vi "Update Graph Plots.vi"(11 "UI Data in":refnum<class "Settings UI.lvclass">) -> (3 "UI Data out":refnum<class "Settings UI.lvclass">)   [LabVIEW 2020, in "Output Sequencer.lvlib" / "Settings UI.lvclass"]
uses:
  Settings UI.lvclass
  Settings UI.lvclass/Settings UI.ctl
  Output Sequencer/Globals/Global Strings.vi
  Output Sequencer/Output Sequencer.lvclass
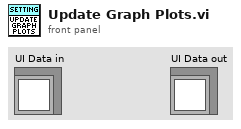
[diagram p1: front panel]
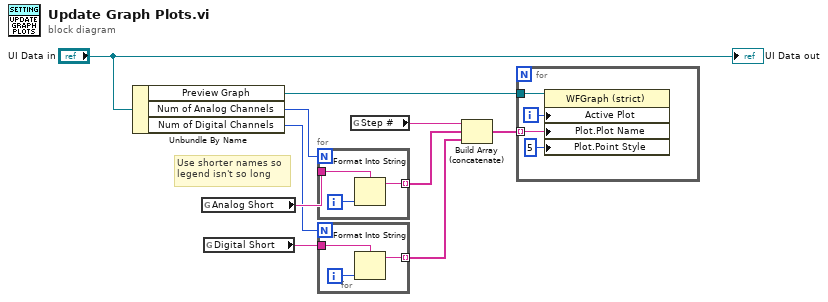
[diagram p0: block diagram]
diagram:
  # "Use shorter names so\nlegend isn't so long"
  n1 = Unbundle By Name("UI Data in") -> ("Preview Graph"=w4:refnum<vi>, "Num of Analog Channels"=w9:i32, "Num of Digital Channels"=w2:i32)
  n2 = global read "Global Strings.vi" "Analog Short"() -> (w5:string)
  n3 = global read "Global Strings.vi" "Digital Short"() -> (w3:string)
  n4 = for {
    N: w9 -> [_]
    tunnel: w5 -> [w12]
    tunnel: [w11] -> w6 mode=indexing
    i -> [w13]
    n5 = Format Into String(format string=w12, w13) -> (resulting string=w11:string)  [unwired: 2 in, 1 out]
  }
  n6 = for {
    N: w2 -> [_]
    tunnel: w3 -> [w15]
    tunnel: [w14] -> w1 mode=indexing
    i -> [w16]
    n7 = Format Into String(format string=w15, w16) -> (resulting string=w14:string)  [unwired: 2 in, 1 out]
  }
  n8 = global read "Global Strings.vi" "Step #"() -> (w7:string)
  n9 = Build Array (concatenate)(w7, w6, w1) -> (w8:string[])
  n10 = for {
    tunnel: w8 -> [w19] mode=indexing
    tunnel: w4 -> [w17]
    i -> [w20]
    n11 = property class="WFGraph (strict)"(reference=w17, "Active Plot"=w20, "Plot.Plot Name"=w19, "Plot.Point Style"=u8 5) -> ()  [unwired: 1 in, 2 out]
  }
  "UI Data out" <- "UI Data in"
